vi "Get Acquired Data.vi"(8 "error in (no error)":errorcluster, 11 "CCDCamera in":refnum<class "iKon-L.lvclass">) -> (0 "error out":errorcluster, 3 "CCDCamera out":refnum<class "iKon-L.lvclass">)   [LabVIEW 2018, in "iKon-L.lvclass"]
doc: "Get the last image acquired by the camera"
uses:
  iKon-L.lvclass
  C:/Users/Denis/Desktop/S4ACS/S4ACS/Sim_CCD/Sim_CCD.lvclass
  Sim_CCD/Sim_CCD.lvclass
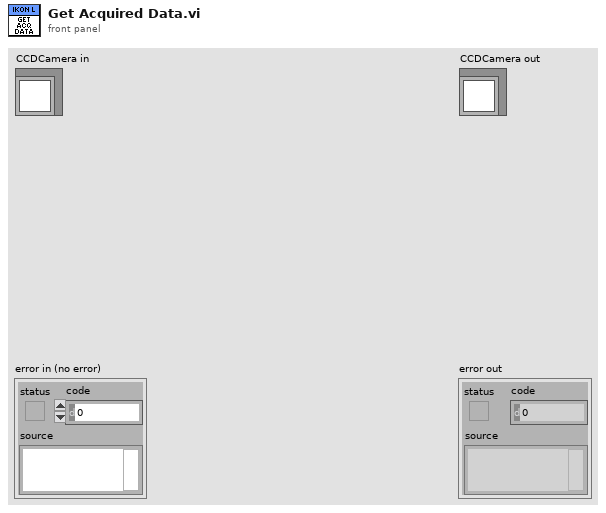
[diagram p1: front panel]
types:
  T1 = cluster{"FRAMES_DONE":u16, "CCD_STATUS":string, "CURRENT_TEMPERATURE":i16, "TEMPERATURE_STATUS":string, "FRAME_EXPOSURE_TIME":dbl, "SERIAL_NUMBER":u16, "ACQUIRING":bool, "POWER":bool, "ACS MODE":bool}
  T2 = cluster{"PREAMP":u16, "READOUT_RATE":u16, "VERTICAL_SHIFT_SPEED":u16, "READ_MODE":u16, "VERTICAL_CLOCK_VOLTAGE":u16, "ACQUISITION_MODE":u16, "AD_CHANNEL":u16, "SHUTTER_TTL":u16, "SHUTTER_OPENING_TIME":u16, "SHUTTER_CLOSING_TIME":u16, "SHUTTER_MODE":u16, "TRIGGER_MODE":u16, "VBIN":u16, "INITIAL_LINE":u16, "INITIAL_COLUMN":u16, "FINAL_LINE":u16, "FINAL_COLUMN":u16, "HBIN":u16}
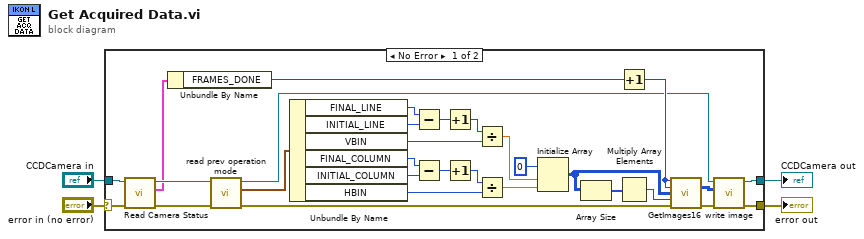
[diagram p0: block diagram]
diagram:
  n1 = case shown="No Error" "error in (no error)" {
    selector: "error in (no error)" -> [w16 w36]
    tunnel: [w6 w36] -> w1
    tunnel: [w5 w35] -> w2
    tunnel: "CCDCamera in" -> [w13 w35]
    frame No Error {
      n2 = call "Read Camera Status.vi"("error in (no error)"=w16, "CCDCamera in"=w13) -> ("error out"=w15:errorcluster, "camera status"=w12:T1, "CCDCamera out"=w14:refnum<class "iKon-L.lvclass">)  [unwired: 7 in]
      n3 = Unbundle By Name(w12) -> ("FRAMES_DONE"=w11:u16)
      n4 = call "read prev operation mode.vi"("error in (no error)"=w15, "Simulated_CCD_Camera in"=w14) -> ("error out"=w18:errorcluster, "prev operation mode"=w17:T2, "Simulated_CCD_Camera out"=w8:refnum<class "iKon-L.lvclass">)  [unwired: 7 in]
      n5 = Unbundle By Name(w17) -> ("FINAL_LINE"=w19:u16, "INITIAL_LINE"=w20:u16, "VBIN"=w21:u16, "FINAL_COLUMN"=w22:u16, "INITIAL_COLUMN"=w23:u16, "HBIN"=w24:u16)
      n6 = Subtract(x=w19, y=w20) -> (x-y=w34:u16)
      n7 = Subtract(x=w22, y=w23) -> (x-y=w33:u16)
      n8 = Increment(x=w34) -> (x+1=w32:u16)
      n9 = Increment(x=w33) -> (x+1=w31:u16)
      n10 = Divide(x=w32, y=w21) -> (x/y=w29:dbl)
      n11 = Divide(x=w31, y=w24) -> (x/y=w28:dbl)
      n12 = Initialize Array(u16 0, w29, w28) -> (w27:u16[][])
      n13 = Array Size(array=w27) -> (size(s)=w26:i32[])
      n14 = Increment(x=w11) -> (x+1=w10:u16)
      n15 = Multiply Array Elements(1:w26) -> (0:w25:i32)
      n16 = call <userlib>:"GetImages16.vi"("first"=w10, "last"=w10, "array"=w27, "size"=w25, "error in (no error)"=w18) -> ("array"=w9:u16[][], "error out"=w7:errorcluster)  [unwired: 6 in, 3 out]
      n17 = call "write image.vi"("error in (no error)"=w7, "Image Graph"=w9, "CCDCamera in"=w8) -> ("error out"=w6:errorcluster, "CCDCamera out"=w5:refnum<class "iKon-L.lvclass">)  [unwired: 7 in]
    }
    frame Error {
    }
  }
  "error out" <- w1
  "CCDCamera out" <- w2
